vi "offline_wavlength_lock.vi"(4 "Device":refnum<visa-resource-name>="Pro8000", 6 "Settings":T2={"Module"=enum."WV Online TEC", "WV Online TEC"=23.169499999999484, "WV Online LD"=0.175, "WV Offline TEC"=29.51225, "WV Offline LD"=0.175, "WV Etalon TEC"=30.4, "HSRL Etalon TEC"=25.954, "HSRL TEC"=14.28699999999974, "HSRL LD"=0.16} {"HSRL LD" min=0.0 max=0.18 step=0.001 format="%.3p"; "HSRL TEC" min=14.0 max=28.0 step=0.1 format="%.3g"; "WV Offline LD" min=0.0 max=0.18 step=0.001 format="%.3p"; "WV Online LD" min=0.0 max=0.18 step=0.001 format="%.3p"; "HSRL Etalon TEC" format="%.2g"; "WV Etalon TEC" format="%.2g"; "WV Offline TEC" min=16.0 max=30.0 step=0.1 format="%.3g"; "WV Online TEC" min=14.0 max=28.0 step=0.1 format="%.3g"}, 7 "Lambda Off Set (nm)":dbl=780.1 format="%.5f", 8 "step_size":dbl=0.0005 format="%#_6p") -> (1 "Wavelength Lock Offline":bool=TRUE, 2 "Lambda Off Read (nm)":dbl=828.2974558529467 format="%.5f")   [LabVIEW 2012]
uses:
  <vilib>/DAQmx/write.llb/DAQmx Write (Digital 1D Bool NChan 1Samp 1Line).vi
  <vilib>/DAQmx/miscellaneous.llb/DAQmx Fill In Error Info.vi
  Shared Telescope WV DIAL Code/bristol/CLDevIFace.dll
panel:
  out "Readings":T1={"Pro8000"=TRUE, "WV OnLine TEC"=23.1755314, "WV Online TEC"=TRUE, "WV Online LD"=0.175443366, "WV Online LD"=TRUE, "WV Offline TEC"=29.5255375, "WV Offline TEC"=TRUE, "WV Offline LD"=0.175283208, "WV Offline LD"=TRUE, "WV EtalonTEC"=30.4229469, "WV Etalon TEC"=TRUE, "HSRL Etalon TEC"=25.9482574, "HSRL Etalon TEC"=TRUE, "HSRL TEC"=14.2977543, "HSRL TEC "=TRUE, "HSRL LD"=0.160093755, "HSRL LD"=TRUE} {"HSRL LD" format="%.3p"; "HSRL TEC" format="%.3g"; "WV Offline LD" format="%.3p"; "WV Online LD" format="%.3p"; "HSRL Etalon TEC" format="%.3g"; "WV EtalonTEC" format="%.3g"; "WV Offline TEC" format="%.3g"; "WV OnLine TEC" format="%.3g"}
  in  "Offline_Tol":dbl=0.0001 format="%#_15g"
  out "WL_Difference":dbl=5.8529466286927345e-06 format="%#_3e"
  in  "Cancel offline":bool
  in  "Bristol In":i32=5
  out "Bristol Out":i32
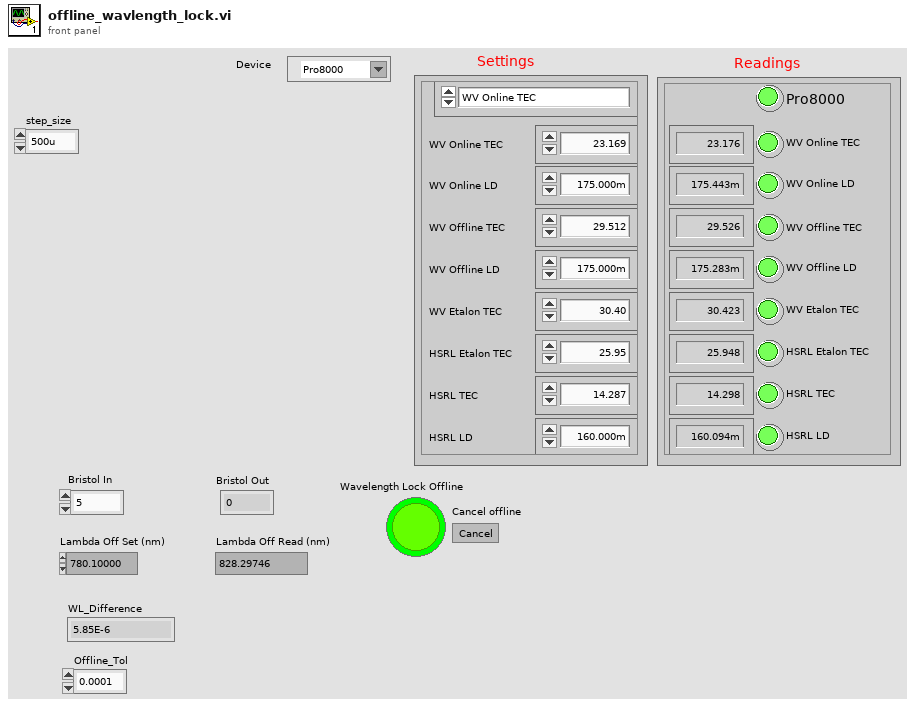
[diagram p1: front panel]
types:
  T1 = cluster{"Pro8000":bool, "WV OnLine TEC":dbl, "WV Online TEC":bool, "WV Online LD":dbl, "WV Online LD":bool, "WV Offline TEC":dbl, "WV Offline TEC":bool, "WV Offline LD":dbl, "WV Offline LD":bool, "WV EtalonTEC":dbl, "WV Etalon TEC":bool, "HSRL Etalon TEC":dbl, "HSRL Etalon TEC":bool, "HSRL TEC":dbl, "HSRL TEC ":bool, "HSRL LD":dbl, "HSRL LD":bool}
  T2 = cluster{"Module":enum16{"WV Online TEC", "WV Online LD", "WV Offline TEC", "WV Offline LD", "WV Etalon TEC", "HSRL Etalon TEC", "HSRL TEC", "HSRL LD"}, "WV Online TEC":dbl, "WV Online LD":dbl, "WV Offline TEC":dbl, "WV Offline LD":dbl, "WV Etalon TEC":dbl, "HSRL Etalon TEC":dbl, "HSRL TEC":dbl, "HSRL LD":dbl}
  T3 = enum16{"WV Online TEC", "WV Online LD", "WV Offline TEC", "WV Offline LD", "WV Etalon TEC", "HSRL Etalon TEC", "HSRL TEC", "HSRL LD"}
  T4 = enum16{"Open_TL", "Close_TL", "Verify_ID", "TEC_Sensor", "SET", "READ", "ON", "OFF", "Set_Limits", "Read_Limits", "Enable_Status", "Read_Status"}
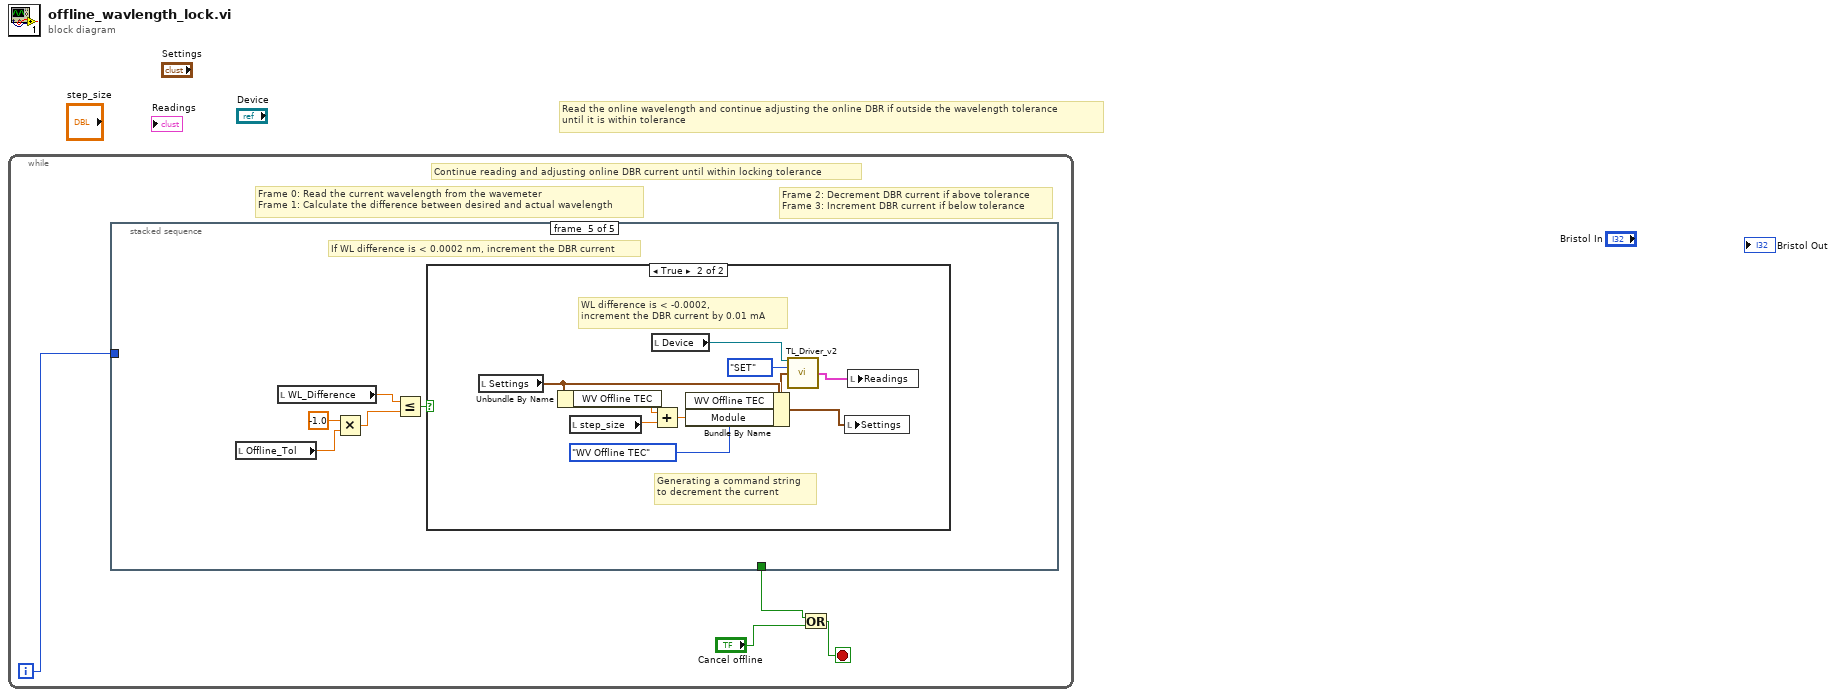
[diagram p0: block diagram]
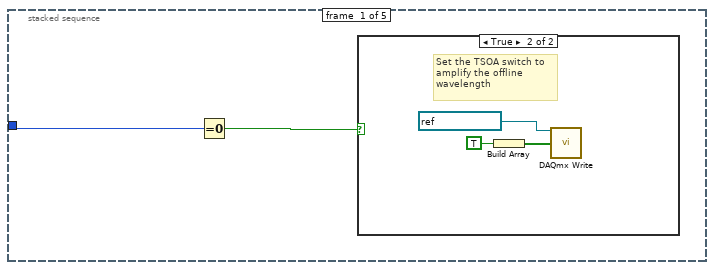
[diagram p2: hidden frame]
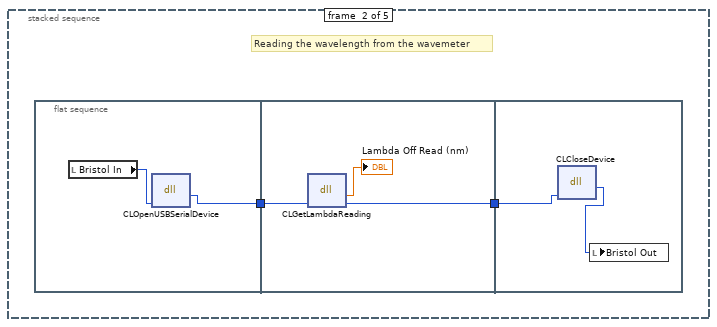
[diagram p4: hidden frame]
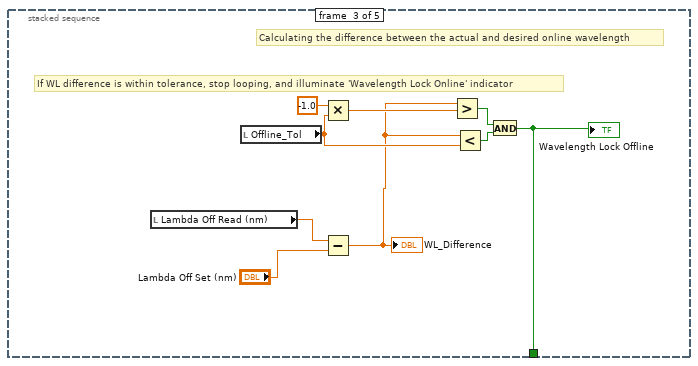
[diagram p5: hidden frame]
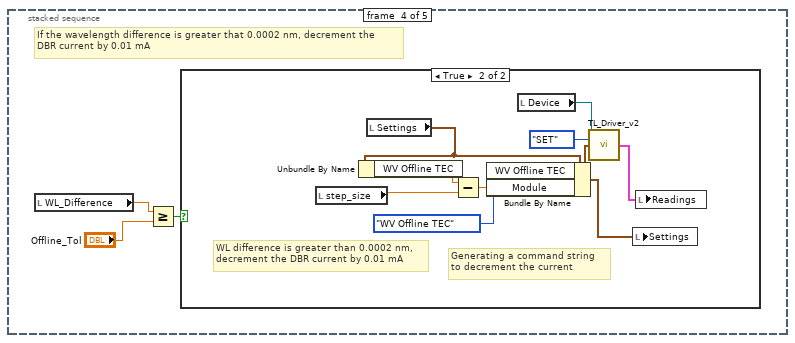
[diagram p6: hidden frame]
diagram:
  # "Read the online wavelength and continue adjusting the online DBR if outside the wavelength tolerance\nuntil it is within tolerance"
  n1 = while {
    i -> [w4]
    stop <- w1 stop-if-true
    # "Frame 2: Decrement DBR current if above tolerance\nFrame 3: Increment DBR current if below tolerance"
    # "Frame 0: Read the current wavelength from the wavemeter\nFrame 1: Calculate the difference between desired and actual wavelength"
    # "Continue reading and adjusting online DBR current until within locking tolerance"
    n2 = stacked-sequence {
      tunnel: w4 -> [w6 _ _ _ _]
      tunnel: [_ _ w19 _ _] -> w2
      frame #0 {
        n3 = Equal To 0?(x=w6) -> (x = 0?=w5:bool)
        n4 = case shown="True" w5 {
          frame False {
          }
          frame True {
            # "Set the TSOA switch to\namplify the offline\nwavelength"
            n5 = Build Array(TRUE ("Boolean")) -> (w7:bool[])
            n6 = call-poly <vilib>:"DAQmx Write.vi"("task/channels in"=refnum<k21> "BristolWM", "data"=w7) -> ()  [unwired: 11 in, 3 out]
          }
        }
      }
      frame #1 {
        # "Reading the wavelength from the wavemeter"
        n7 = flat-sequence {
          tunnel: [w12] -> w11
          tunnel: w11 -> [w15]
          tunnel: [w14] -> w10
          tunnel: w10 -> [w18]
          frame #0 {
            n8 = local read "Bristol In"() -> (w13:i32)
            n9 = dll-call lib="C:/Users/H2ODial/Desktop/Shared Telescope WV DIAL Code/bristol/CLDevIface.dll" fn="CLOpenUSBSerialDevice"("commPort"=w13) -> ("return type"=w12:i32)  [unwired: 4 in, 2 out]
          }
          frame #1 {
            n10 = dll-call lib="C:/Users/H2ODial/Desktop/Shared Telescope WV DIAL Code/bristol/CLDevIface.dll" fn="CLGetLambdaReading"("devHandle"=w15) -> ("return type"=→"Lambda Off Read (nm)":dbl, "devHandle"=w14:i32)  [unwired: 3 in, 2 out]
          }
          frame #2 {
            n11 = dll-call lib="C:/Users/H2ODial/Desktop/Shared Telescope WV DIAL Code/bristol/CLDevIface.dll" fn="CLCloseDevice"("commPort"=w18) -> ("return type"=w17:i32)  [unwired: 4 in, 2 out]
            n12 = local write "Bristol Out"(w17) -> ()
          }
        }
      }
      frame #2 {
        # "If WL difference is within tolerance, stop looping, and illuminate 'Wavelength Lock Online' indicator"
        # "Calculating the difference between the actual and desired online wavelength"
        n13 = local read "Lambda Off Read (nm)"() -> (w27:dbl)
        n14 = local read "Offline_Tol"() -> (w24:dbl)
        n15 = Multiply(x=-1.0, y=w24) -> (x*y=w25:dbl)
        n16 = Subtract(x=w27, y="Lambda Off Set (nm)") -> (x-y=w20:dbl)
        "WL_Difference" <- w20
        n17 = Greater?(x=w20, y=w25) -> (0:w21:bool)
        n18 = Less?(x=w20, y=w24) -> (x < y?=w22:bool)
        n19 = And(x=w21, y=w22) -> (x .and. y?=w19:bool)
        "Wavelength Lock Offline" <- w19
      }
      frame #3 {
        # "If the wavelength difference is greater that 0.0002 nm, decrement the \nDBR current by 0.01 mA"
        n20 = local read "WL_Difference"() -> (w30:dbl)
        n21 = Greater Or Equal?(x=w30, y="Offline_Tol") -> (x >= y?=w29:bool)
        n22 = case shown="True" w29 {
          frame False {
            # "Wavelength difference is not greater than 0.0002 nm, do nothing"
          }
          frame True {
            # "Generating a command string\nto decrement the current"
            # "WL difference is greater than 0.0002 nm,\ndecrement the DBR current by 0.01 mA"
            n23 = local read "step_size"() -> (w36:dbl)
            n24 = local read "Settings"() -> (w35:T2)
            n25 = Unbundle By Name(w35) -> ("WV Offline TEC"=w39:dbl)
            n26 = Subtract(x=w39, y=w36) -> (x-y=w38:dbl)
            n27 = Bundle By Name(cluster=w35, "WV Offline TEC"=w38, "Module"=T3."WV Offline TEC") -> (w31:T2)
            n28 = local read "Device"() -> (w34:refnum<visa-resource-name>)
            n29 = call "TL_Driver_v2.vi"("Device In"=w34, "Commands"=T4."SET", "Settings"=w31) -> ("Readings"=w33:T1)  [unwired: 9 in, 3 out]
            n30 = local write "Settings"(w31) -> ()
            n31 = local write "Readings"(w33) -> ()
          }
        }
      }
      frame #4 {
        # "If WL difference is < 0.0002 nm, increment the DBR current"
        n32 = local read "Offline_Tol"() -> (w41:dbl)
        n33 = local read "WL_Difference"() -> (w44:dbl)
        n34 = Multiply(x=-1.0, y=w41) -> (x*y=w40:dbl)
        n35 = Less Or Equal?(x=w44, y=w40) -> (x <= y?=w43:bool)
        n36 = case shown="True" w43 {
          frame False {
            # "WL difference is no <= to -0.0002 nm, do nothing"
          }
          frame True {
            # "WL difference is < -0.0002,\nincrement the DBR current by 0.01 mA"
            # "Generating a command string\nto decrement the current"
            n37 = local read "Settings"() -> (w53:T2)
            n38 = Unbundle By Name(w53) -> ("WV Offline TEC"=w51:dbl)
            n39 = local read "step_size"() -> (w47:dbl)
            n40 = local read "Device"() -> (w48:refnum<visa-resource-name>)
            n41 = Add(x=w51, y=w47) -> (x+y=w50:dbl)
            n42 = Bundle By Name(cluster=w53, "WV Offline TEC"=w50, "Module"=T3."WV Offline TEC") -> (w45:T2)
            n43 = call "TL_Driver_v2.vi"("Device In"=w48, "Commands"=T4."SET", "Settings"=w45) -> ("Readings"=w46:T1)  [unwired: 9 in, 3 out]
            n44 = local write "Settings"(w45) -> ()
            n45 = local write "Readings"(w46) -> ()
          }
        }
      }
    }
    n46 = Or(x=w2, y="Cancel offline") -> (x .or. y?=w1:bool)
  }
